vi "ReadRightData.vi"(6 "timeout in ms (-1)":i32, 8 "error in (no error)":errorcluster, 11 "MAUI in":refnum<class "MAUI.lvclass">) -> (0 "error out":errorcluster, 2 "Right":T1, 3 "MAUI out":refnum<class "MAUI.lvclass">)   [LabVIEW 2016]
uses:
  MAUI.lvclass
  Typedefs/PanelData.ctl
  Typedefs/PrivateEvents--MAUI.GetRightData.ctl
  C:/Program Files (x86)/National Instruments/LabVIEW 2016/vi.lib/JKI/JKI SMO/SMO.UI/SMO.UI.lvclass
  C:/Program Files (x86)/National Instruments/LabVIEW 2016/vi.lib/JKI/JKI SMO/SMO/SMO.lvclass
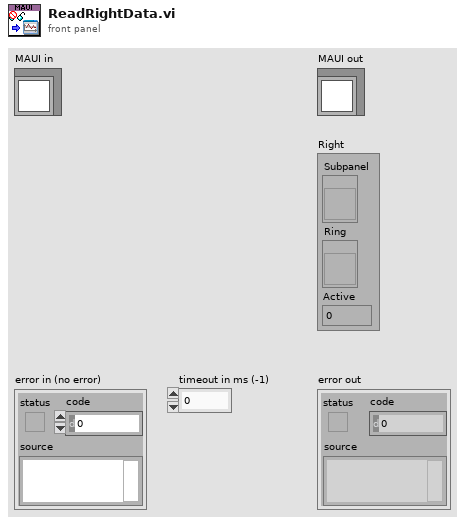
[diagram p1: front panel]
types:
  T1 = typedef "MAUI.lvclass/PanelData.ctl" = cluster{"Subpanel":refnum<vi>, "Ring":refnum<vi>, "Active":i32}
  T2 = typedef "MAUI.lvclass/PrivateEvents--MAUI.GetRightData.ctl" = cluster{"notifier":refnum<notifier>}
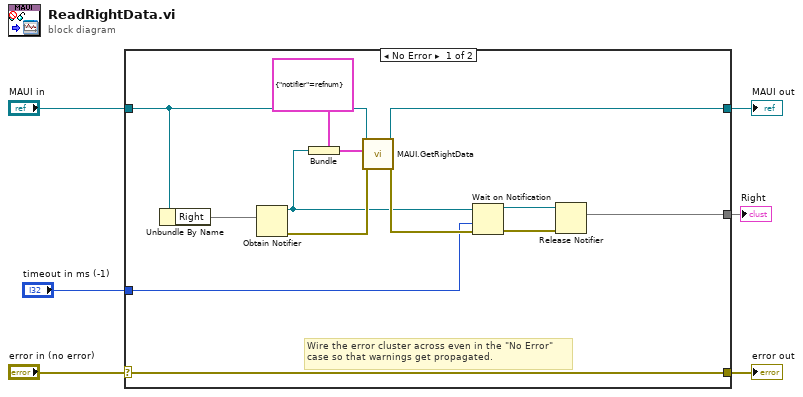
[diagram p0: block diagram]
diagram:
  n1 = case shown="No Error" "error in (no error)" {
    selector: "error in (no error)" -> [w19 w21]
    tunnel: [w19 w21] -> w5
    tunnel: [w7 w20] -> w3
    tunnel: "MAUI in" -> [w8 w20]
    tunnel: "timeout in ms (-1)" -> [w12 _]
    tunnel: [w9 _] -> w1
    frame No Error {
      # "Wire the error cluster across even in the \"No Error\"\ncase so that warnings get propagated."
      n2 = Unbundle By Name(w8) -> ("Right"=w18)
      n3 = Obtain Notifier(notification data type=w18) -> (notifier out=w13:refnum<notifier>, error out=w15:errorcluster)  [unwired: 3 in, 1 out]
      n4 = Bundle(cluster=T2 {"notifier"=refnum} ("GetRightData"), "notifier"=w13) -> (w16:T2)
      n5 = call "MAUI.GetRightData.vi"("error in (no error)"=w15, "GetRightData"=w16, "MAUI"=w8) -> ("error out"=w14:errorcluster, "MAUI out"=w7:refnum<class "MAUI.lvclass">)  [unwired: 7 in]
      n6 = Wait on Notification(notifier=w13, timeout in ms (-1)=w12, error in (no error)=w14) -> (notifier out=w11:refnum<notifier>, error out=w10:errorcluster)  [unwired: 1 in, 2 out]
      n7 = Release Notifier(notifier=w11, error in (no error)=w10) -> (last notification=w9)  [unwired: 1 in, 2 out]
    }
    frame Error {
    }
  }
  "error out" <- w5
  "MAUI out" <- w3
  "Right" <- w1
